vi "LVIS_LaunchStatus.vi"(8 "Error In":errorcluster) -> (0 "Error Out":errorcluster)   [LabVIEW 2015]
doc: "Launches the Status process responsible for polling the Data Commander SAF state."
uses:
  Globals/LVIS_IsGlobal.vi
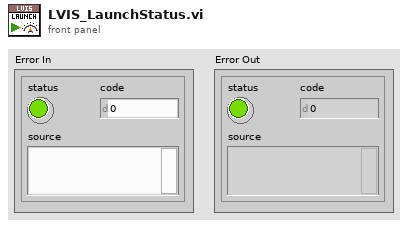
[diagram p1: front panel]
types:
  T1 = enum32{"Invalid", "Standard", "Closed", "Hidden", "Minimized", "Maximized"}
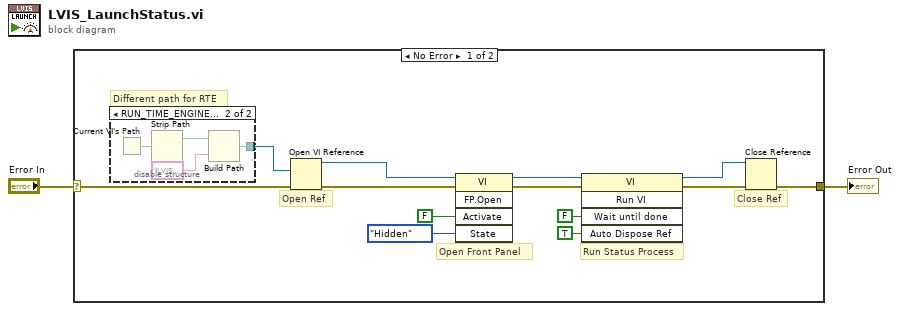
[diagram p0: block diagram]
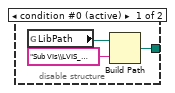
[diagram p2: hidden frame]
diagram:
  n1 = case shown="No Error" "Error In" {
    selector: "Error In" -> [w15 w23]
    tunnel: [w14 w23] -> w1
    frame No Error {
      # "Different path for RTE"
      # "Open Ref"
      # "Run Status Process"
      # "Open Front Panel"
      # "Close Ref"
      n2 = disable-structure shown="RUN_TIME_ENGINE==True" {
        disable-tunnel: [w16 w19] -> w3
        frame condition #0 (active) {
          n3 = global read "LVIS_IsGlobal.vi" "LibPath"() -> (w18:path)
          n4 = Build Path(base path=w18, name or relative path="Sub VIs\\LVIS_Status.vi") -> (appended path=w16:path)
        }
        frame condition #1 {
          n5 = Current VI's Path() -> (path=w22:path)
          n6 = Strip Path(path=w22) -> (stripped path=w21:path)  [unwired: 1 out]
          n7 = Build Path(base path=w21, name or relative path="LVIS_Status.vi") -> (appended path=w19:path)
        }
      }
      n8 = Open VI Reference(vi path=w3, error in (no error)=w15) -> (vi reference=w4:refnum<vi>, error out=w5:errorcluster)  [unwired: 4 in]
      n9 = invoke class="VI" method="FP.Open"(reference=w4, error in=w5, "Activate"=FALSE ("Activate?"), "State"=T1."Hidden") -> (reference out=w8:refnum<vi>, error out=w9:errorcluster)  [unwired: 1 in, 3 out]
      n10 = invoke class="VI" method="Run VI"(reference=w8, error in=w9, "Wait until done"=FALSE ("Wait Until Done"), "Auto Dispose Ref"=TRUE ("Auto Dispose Reference")) -> (reference out=w12:refnum<vi>, error out=w13:errorcluster)  [unwired: 1 in, 3 out]
      n11 = Close Reference(reference=w12, error in (no error)=w13) -> (error out=w14:errorcluster)
    }
    frame Error {
    }
  }
  "Error Out" <- w1
